vi "Joystick Sensitivity Test.vi"(7 "Bypass Joystick Sensitivity":bool, 8 "Turn Throtle (0 to +1)":dbl min=0.0 max=1.0 step=0.1 format="%#_5g", 9 "Turn Joystick Output (-1 to +1)":dbl min=-1.0 max=1.0 step=0.1 format="%#_5g", 10 "Speed Throtle (0 to +1)":dbl min=0.0 max=1.0 step=0.1 format="%#_5g", 11 "Speed Joystick Output (-1 to +1)":dbl min=-1.0 max=1.0 step=0.1 format="%#_5g") -> (2 "Turn Sensitivity Adjusted Output (-1 to +1)":dbl min=-1.0 max=1.0 format="%#_5g", 3 "Speed Sensitivity Adjusted Output (-1 to +1)":dbl min=-1.0 max=1.0 format="%#_5g")   [LabVIEW 2017]
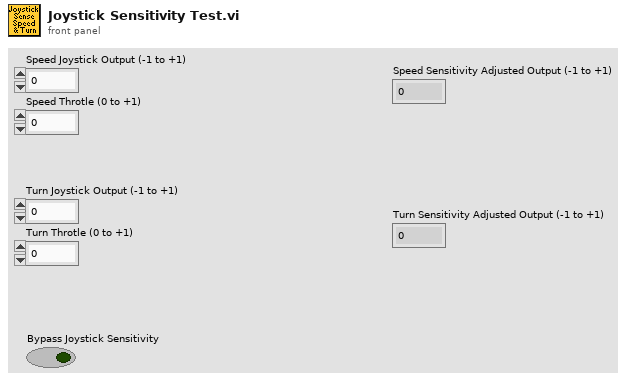
[diagram p1: front panel]
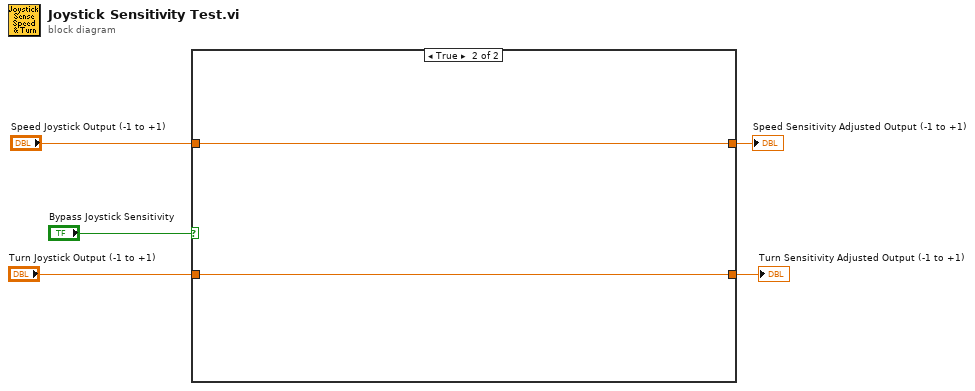
[diagram p0: block diagram]
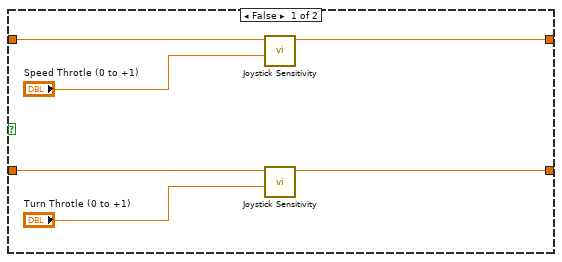
[diagram p2: hidden frame]
diagram:
  n1 = case shown="True" "Bypass Joystick Sensitivity" {
    tunnel: "Speed Joystick Output (-1 to +1)" -> [w9 w13]
    tunnel: "Turn Joystick Output (-1 to +1)" -> [w8 w12]
    tunnel: [w7 w13] -> w2
    tunnel: [w6 w12] -> w1
    frame False {
      n2 = call "Joystick Sensitivity.vi"("Throtle (0 to +1)"="Speed Throtle (0 to +1)", "Joystick Output (-1 to +1)"=w9) -> ("Sensitivity Adjusted Output (-1 to +1)"=w7:dbl)  [unwired: 9 in]
      n3 = call "Joystick Sensitivity.vi"("Throtle (0 to +1)"="Turn Throtle (0 to +1)", "Joystick Output (-1 to +1)"=w8) -> ("Sensitivity Adjusted Output (-1 to +1)"=w6:dbl)  [unwired: 9 in]
    }
    frame True {
    }
  }
  "Speed Sensitivity Adjusted Output (-1 to +1)" <- w2
  "Turn Sensitivity Adjusted Output (-1 to +1)" <- w1
